vi "plot magnetotropic -- all.vi"() -> ()   [LabVIEW 2020]
uses:
  <vilib>/event_ctls.llb/eventvkey.ctl
  <vilib>/Analysis/baseanly.llb/A x Vector.vi
  <vilib>/Analysis/baseanly.llb/Complex A x B.vi
  Q -- check range -- i -- real.vi
  line -- complex.vi
  Q -- check range -- i -- integer.vi
  aggregator - v - real - atomic.vi
  Q - not nan -- real.vi
  Q - not nan -- integer.vi
  linear interpolation - real.vi
  <vilib>/Analysis/Matrix/Numeric/Conversions/Array To Matrix.vi
  <vilib>/Analysis/Matrix/Numeric/Conversions/Array To Matrix - RA2.vi
  <vilib>/Analysis/baseanly.llb/Inverse Matrix.vi
  <vilib>/Analysis/baseanly.llb/Real Inverse Matrix.vi
  <vilib>/Analysis/NI_AALBase.lvlib
panel:
  in  "Tab Control":enum32{"Page 1", "Page 2"}(tab)
  in  "max alpha":dbl=360.0 format="%#_13g"
  out "Plot angles":cluster{dbl[], dbl[]}[](graph)=[{[0.0, 3.6, 7.2, 10.8, 14.4, 18.0, 21.6, 25.2, 28.8, 32.4, 36.0, 39.6, 43.2, 46.800000000000004, 50.4, 54.0, 57.6, 61.2, 64.8, 68.4, 72.0, 75.60000000000001, 79.2, 82.8, 86.4, 90.0, 93.60000000000001, 97.2, 100.8, 104.4, 108.0, 111.60000000000001, 115.2, 118.8, 122.4, 126.0, 129.6, 133.20000000000002, 136.8, 140.4, 144.0, 147.6, 151.20000000000002, 154.8, 158.4, 162.0, 165.6, 169.20000000000002, 172.8, 176.4, 180.0, 183.6, 187.20000000000002, 190.8, 194.4, 198.0, 201.6, 205.20000000000002, 208.8, 212.4, 216.0, 219.6, 223.20000000000002, 226.8, 230.4, 234.0, 237.6, 241.20000000000002, 244.8, 248.4, 252.0, 255.6, 259.2, 262.8, 266.40000000000003, 270.0, 273.6, 277.2, 280.8, 284.40000000000003, 288.0, 291.6, 295.2, 298.8, 302.40000000000003, 306.0, 309.6, 313.2, 316.8, 320.40000000000003, 324.0, 327.6, 331.2, 334.8, 338.40000000000003, 342.0, 345.6, 349.2, 352.8, 356.40000000000003], [-313.48146927140203, -305.858243348933, -284.2953550420243, -252.19459672026446, -213.84280315872593, -173.21720232347388, -133.2937756788047, -95.90672651415247, -61.945212185027714, -31.65615222148574, -4.916123418277465, 18.574327400526585, 39.170983826139434, 57.2211441404977, 73.03368491463019, 86.86906141407903, 98.9396043298828, 109.4144526814921, 118.42604419322804, 126.07661803927712, 132.44403837415837, 137.5866937086247, 141.54744356495215, 144.3566756438778, 146.03456403347786, 146.59261453117998, 146.03456403347747, 144.35667564387575, 141.54744356495738, 137.58669370862123, 132.4440383741633, 126.07661803929162, 118.42604419322953, 109.4144526814938, 98.93960432990127, 86.86906141404705, 73.03368491462109, 57.22114414049983, 39.170983826133465, 18.574327400523742, -4.916123418274623, -31.65615222148702, -61.945212185040646, -95.90672651414792, -133.29377567881153, -173.2172023234709, -213.84280315872715, -252.19459672026204, -284.29535504202454, -305.8582433489345, -313.4814692714306, -305.85824334893397, -284.2953550420227, -252.19459672026284, -213.84280315872985, -173.21720232347118, -133.29377567881508, -95.90672651414764, -61.9452121850415, -31.65615222148702, -4.916123418278744, 18.5743274005182, 39.170983826133465, 57.22114414047297, 73.0336849146181, 86.86906141404975, 98.93960432989743, 109.41445268149444, 118.42604419322932, 126.07661803929105, 132.44403837416343, 137.58669370862128, 141.54744356495735, 144.35667564387546, 146.03456403347747, 146.59261453117998, 146.03456403347553, 144.3566756438778, 141.54744356495374, 137.58669370862498, 132.4440383741574, 126.07661803927712, 118.42604419322853, 109.41445268148918, 98.93960432988536, 86.86906141408315, 73.03368491460375, 57.2211441404977, 39.1709838261356, 18.574327400526585, -4.916123418277465, -31.656152221493272, -61.945212185025866, -95.90672651419283, -133.29377567880485, -173.21720232347545, -213.84280315872545, -252.19459672026517, -284.29535504202306, -305.85824334893294]}, {[0.0, 3.6, 7.2, 10.8, 14.4, 18.0, 21.6, 25.2, 28.8, 32.4, 36.0, 39.6, 43.2, 46.800000000000004, 50.4, 54.0, 57.6, 61.2, 64.8, 68.4, 72.0, 75.60000000000001, 79.2, 82.8, 86.4, 90.0, 93.60000000000001, 97.2, 100.8, 104.4, 108.0, 111.60000000000001, 115.2, 118.8, 122.4, 126.0, 129.6, 133.20000000000002, 136.8, 140.4, 144.0, 147.6, 151.20000000000002, 154.8, 158.4, 162.0, 165.6, 169.20000000000002, 172.8, 176.4, 180.0, 183.6, 187.20000000000002, 190.8, 194.4, 198.0, 201.6, 205.20000000000002, 208.8, 212.4, 216.0, 219.6, 223.20000000000002, 226.8, 230.4, 234.0, 237.6, 241.20000000000002, 244.8, 248.4, 252.0, 255.6, 259.2, 262.8, 266.40000000000003, 270.0, 273.6, 277.2, 280.8, 284.40000000000003, 288.0, 291.6, 295.2, 298.8, 302.40000000000003, 306.0, 309.6, 313.2, 316.8, 320.40000000000003, 324.0, 327.6, 331.2, 334.8, 338.40000000000003, 342.0, 345.6, 349.2, 352.8, 356.40000000000003], [-52.098103078947666, -64.89098767355117, -109.04888534951418, -194.42645181689528, -298.8059333429718, -335.9390833991341, -266.9407778689754, -169.02628156661706, -97.14690185514655, -50.71491152292708, -18.003664188575215, 7.871623107547521, 29.77997548820923, 48.851124152969874, 65.59614496908608, 80.3111497772457, 93.20434301282972, 104.4349357297611, 114.1270103434394, 122.37670334950465, 129.25744555823945, 134.82430138343324, 139.11757735713303, 142.16571872494595, 143.98751207706195, 144.5936246043267, 143.98751207706334, 142.16571872494666, 139.1175773571345, 134.8243013834304, 129.2574455582536, 122.37670334947296, 114.12701034343726, 104.4349357297638, 93.2043430128337, 80.31114977728095, 65.59614496910967, 48.85112415302615, 29.77997548822117, 7.871623107423034, -18.00366418848654, -50.71491152304105, -97.14690185523153, -169.02628156654373, -266.9407778689721, -335.93908339917783, -298.8059333429725, -194.42645181688215, -109.0488853495065, -64.89098767354592, -52.09810307894766, -64.89098767354581, -109.04888534950685, -194.42645181688349, -298.80593334297214, -335.93908339917874, -266.94077786899186, -169.0262815665497, -97.14690185522329, -50.71491152305839, -18.003664188560435, 7.87162310743895, 29.77997548822117, 48.85112415304576, 65.59614496911792, 80.31114977728436, 93.20434301282688, 104.43493572977161, 114.12701034343144, 122.37670334946948, 129.25744555825858, 134.82430138342897, 139.11757735713473, 142.16571872494666, 143.98751207706334, 144.59362460432672, 143.9875120770618, 142.16571872494595, 139.11757735713337, 134.82430138343773, 129.25744555823934, 122.37670334949264, 114.12701034342888, 104.43493572976237, 93.20434301284024, 80.31114977723888, 65.59614496908722, 48.851124152969874, 29.779975488203547, 7.871623107547521, -18.003664188575215, -50.71491152291799, -97.14690185517213, -169.02628156661962, -266.9407778689721, -335.93908339913344, -298.80593334296805, -194.42645181689522, -109.04888534951428, -64.89098767355122]}]
  out "weight -- one spin":dbl=-52.99873886913457
  out "weight -- bipartite":dbl=-50.9668248690652
  in  "field":dbl(slide)=100.0 scale=0.0..100.0
  out "Plot":cluster{dbl[], dbl[]}[](graph)=[{[0.0, 2.0, 4.0, 6.0, 8.0, 10.0, 12.0, 14.0, 16.0, 18.0, 20.0, 22.0, 24.0, 26.0, 28.0, 30.0, 32.0, 34.0, 36.0, 38.0, 40.0, 42.0, 44.0, 46.0, 48.0, 50.0, 52.0, 54.0, 56.0, 58.0, 60.0, 62.0, 64.0, 66.0, 68.0, 70.0, 72.0, 74.0, 76.0, 78.0, 80.0, 82.0, 84.0, 86.0, 88.0, 90.0, 92.0, 94.0, 96.0, 98.0, 100.0, 102.0, 104.0, 106.0, 108.0, 110.0, 112.0, 114.0, 116.0, 118.0, 120.0, 122.0, 124.0, 126.0, 128.0, 130.0, 132.0, 134.0, 136.0, 138.0, 140.0, 142.0, 144.0, 146.0, 148.0, 150.0, 152.0, 154.0, 156.0, 158.0, 160.0, 162.0, 164.0, 166.0, 168.0, 170.0, 172.0, 174.0, 176.0, 178.0, 180.0, 182.0, 184.0, 186.0, 188.0, 190.0, 192.0, 194.0, 196.0, 198.0], [0.0, 1.1385133282404225, 3.9788841114054527, 7.490878120034998, 11.038654301749444, 14.427008958566468, 17.658021528651247, 20.779726830573175, 23.83474181657537, 26.851283092850977, 29.845953470720342, 32.82793129135691, 35.802100017435976, 38.77099118470959, 41.73589205829657, 44.69744710271395, 47.655974462149786, 50.61162883821093, 53.56448394311787, 56.514573698509345, 59.46191264750393, 62.40650591614422, 65.34835410385297, 68.2874556359068, 71.22380789870721, 74.15740778407016, 77.0882519491738, 80.01633694023977, 82.94165925124416, 85.86421535166762, 88.78400169961012, 91.7010147479711, 94.61525094734984, 97.52670674741232, 100.43537859753108, 103.3412629471093, 106.24435624570754, 109.14465494316207, 112.04215548948886, 114.93685433509711, 117.82874793066647, 120.71783272722843, 123.60410517612117, 126.48756172904706, 129.36819883805785, 132.246012955557, 135.1210005343324, 137.99315802753523, 140.86248188871986, 143.72896857181993, 146.59261453117998, 149.4534162215584, 152.31137009813247, 155.1664726165046, 158.01872023271412, 160.86810940324898, 163.71463658505473, 166.5582982355258, 169.39909081253347, 172.23701077443422, 175.0720545800654, 177.9042186887598, 180.73349956035088, 183.5598936551813, 186.38339743413349, 189.2040073585988, 192.02171989050532, 194.83653149232848, 197.64843862711643, 200.45743775844693, 203.2635253504933, 206.0666978679967, 208.86695177628366, 211.66428354127544, 214.45868962950044, 217.2501665080932, 220.03871064481868, 222.82431850806068, 225.60698656683422, 228.38671129080834, 231.1634891502969, 233.937316616298, 236.70819016043666, 239.4761062550522, 242.24106137315607, 245.003051988445, 247.7620745753361, 250.51812560894987, 253.27120156510438, 256.02129892038096, 258.7684141520641, 261.5125437382003, 264.2536841575947, 266.9918318897845, 269.7269834150807, 272.4591352145985, 275.1882837702045, 277.9144255645732, 280.637557081188, 283.3576748043006]}, {[0.0, 2.0, 4.0, 6.0, 8.0, 10.0, 12.0, 14.0, 16.0, 18.0, 20.0, 22.0, 24.0, 26.0, 28.0, 30.0, 32.0, 34.0, 36.0, 38.0, 40.0, 42.0, 44.0, 46.0, 48.0, 50.0, 52.0, 54.0, 56.0, 58.0, 60.0, 62.0, 64.0, 66.0, 68.0, 70.0, 72.0, 74.0, 76.0, 78.0, 80.0, 82.0, 84.0, 86.0, 88.0, 90.0, 92.0, 94.0, 96.0, 98.0, 100.0, 102.0, 104.0, 106.0, 108.0, 110.0, 112.0, 114.0, 116.0, 118.0, 120.0, 122.0, 124.0, 126.0, 128.0, 130.0, 132.0, 134.0, 136.0, 138.0, 140.0, 142.0, 144.0, 146.0, 148.0, 150.0, 152.0, 154.0, 156.0, 158.0, 160.0, 162.0, 164.0, 166.0, 168.0, 170.0, 172.0, 174.0, 176.0, 178.0, 180.0, 182.0, 184.0, 186.0, 188.0, 190.0, 192.0, 194.0, 196.0, 198.0], [0.0, 8.900130425564837e-10, 4.980541071344847e-09, 1.8027194455800313e-08, 5.5968542752720894e-08, 1.603846822900161e-07, 4.3714180784073774e-07, 1.1513864569353502e-06, 2.9587779768584587e-06, 7.464085178354467e-06, 1.8562061001715787e-05, 4.5638678412783686e-05, 0.00011117792754096806, 0.0002687627106131862, 0.0006455171293070279, 0.00154184819773502, 0.0036651375561248143, 0.008675688934056123, 0.020458309058919093, 0.04807318354057271, 0.11256725639316362, 0.2625492229354917, 0.609136878749996, 1.401214132611615, 3.1726654095564144, 6.965349415930417, 14.418812324214018, 26.980292311505405, 43.74223661144523, 60.66714990650701, 74.0508267865482, 83.2603048838894, 89.49849983930051, 94.05036922442446, 97.74224194918389, 101.01638492343656, 104.09155006689397, 107.0721685756904, 110.00728703682107, 112.91976128369079, 115.8202004532285, 118.71351867786251, 121.60198947594043, 124.48666403616657, 127.36802830740446, 130.24630699257403, 133.12160404575195, 135.99396755810986, 138.8634197099153, 141.72997059496893, 144.5936246043267, 147.45438337876269, 150.3122471791845, 153.16721552756238, 156.0192875109634, 158.86846192981622, 161.71473737360589, 164.5581122624082, 167.39858487224797, 170.2361533521153, 173.07081573690914, 175.9025699578329, 178.73141385126098, 181.55734516654846, 184.3803615729486, 187.2004606659003, 190.01763997262435, 192.83189695733006, 195.64322902584985, 198.45163352995888, 201.2571077712471, 204.0596490047167, 206.85925444206575, 209.65592125469044, 212.4496465764564, 215.2404275062642, 218.02826111037606, 220.81314442459785, 223.59507445624843, 226.37404818606007, 229.15006256984785, 231.9231145401189, 234.6932010075055, 237.460318862166, 240.2244649750537, 242.9856361990703, 245.74382937016685, 248.49904130838834, 251.25126881880405, 254.0005086923912, 256.7467577068962, 259.4900126275882, 262.2302702079803, 264.96752719051915, 267.70178030720695, 270.433026280264, 273.16126182257307, 275.88648363830816, 278.6086884233937, 281.32787286592304]}, {[0.0, 2.0, 4.0, 6.0, 8.0, 10.0, 12.0, 14.0, 16.0, 18.0, 20.0, 22.0, 24.0, 26.0, 28.0, 30.0, 32.0, 34.0, 36.0, 38.0, 40.0, 42.0, 44.0, 46.0, 48.0, 50.0, 52.0, 54.0, 56.0, 58.0, 60.0, 62.0, 64.0, 66.0, 68.0, 70.0, 72.0, 74.0, 76.0, 78.0, 80.0, 82.0, 84.0, 86.0, 88.0, 90.0, 92.0, 94.0, 96.0, 98.0, 100.0, 102.0, 104.0, 106.0, 108.0, 110.0, 112.0, 114.0, 116.0, 118.0, 120.0, 122.0, 124.0, 126.0, 128.0, 130.0, 132.0, 134.0, 136.0, 138.0, 140.0, 142.0, 144.0, 146.0, 148.0, 150.0, 152.0, 154.0, 156.0, 158.0, 160.0, 162.0, 164.0, 166.0, 168.0, 170.0, 172.0, 174.0, 176.0, 178.0, 180.0, 182.0, 184.0, 186.0, 188.0, 190.0, 192.0, 194.0, 196.0, 198.0], [4.1407275882666, 6.99010825547407, 9.83948892268154, 12.68886958988901, 15.538250257096479, 18.38763092430395, 21.23701159151142, 24.086392258718888, 26.935772925926358, 29.785153593133828, 32.6345342603413, 35.48391492754877, 38.33329559475624, 41.18267626196371, 44.032056929171176, 46.881437596378646, 49.730818263586116, 52.580198930793586, 55.429579598001055, 58.278960265208525, 61.128340932415995, 63.977721599623464, 66.82710226683093, 69.6764829340384, 72.52586360124587, 75.37524426845334, 78.22462493566081, 81.07400560286828, 83.92338627007575, 86.77276693728322, 89.62214760449069, 92.47152827169816, 95.32090893890563, 98.1702896061131, 101.01967027332057, 103.86905094052804, 106.71843160773551, 109.56781227494298, 112.41719294215045, 115.26657360935792, 118.11595427656539, 120.96533494377286, 123.81471561098033, 126.6640962781878, 129.51347694539527, 132.36285761260274, 135.2122382798102, 138.06161894701768, 140.91099961422515, 143.76038028143262, 146.6097609486401, 149.45914161584756, 152.30852228305503, 155.1579029502625, 158.00728361746997, 160.85666428467744, 163.7060449518849, 166.55542561909238, 169.40480628629984, 172.25418695350731, 175.10356762071478, 177.95294828792225, 180.80232895512972, 183.6517096223372, 186.50109028954466, 189.35047095675213, 192.1998516239596, 195.04923229116707, 197.89861295837454, 200.747993625582, 203.59737429278948, 206.44675495999695, 209.29613562720442, 212.1455162944119, 214.99489696161936, 217.84427762882683, 220.6936582960343, 223.54303896324177, 226.39241963044924, 229.2418002976567, 232.09118096486418, 234.94056163207165, 237.78994229927912, 240.6393229664866, 243.48870363369406, 246.33808430090153, 249.187464968109, 252.03684563531647, 254.88622630252394, 257.7356069697314, 260.5849876369389, 263.43436830414635, 266.2837489713538, 269.1331296385613, 271.98251030576876, 274.8318909729762, 277.6812716401837, 280.53065230739116, 283.38003297459863, 286.2294136418061]}]
  in  "g":dbl[](array[numeric])=[2.0, 2.0, 1.0]
  in  "theta v":dbl(slide)=90.0 scale=0.0..180.0
  in  "phi v":dbl(slide)=90.0 scale=-180.0..180.0
  in  "theta r":dbl(slide)=90.0 scale=0.0..180.0
  in  "phi r":dbl(slide)=90.0 scale=-180.0..180.0
  in  "theta 0":dbl(slide) scale=0.0..180.0
  in  "phi 0":dbl(slide)=41.53846153846155 scale=-180.0..180.0
  in  "nsteps":i32=100
  in  "integration nsteps":i32=300
  in  "scale":dbl(slide)=175.50446715591082 scale=0.01..200.0
  in  "alpha":dbl(slide)=90.0 scale=0.0..180.0
  in  "temperature":dbl(slide)=10.0 scale=0.0..300.0
  in  "max B":dbl=200.0 format="%#_13g"
  in  "JR":dbl(slide)=30.0 scale=-100.0..100.0
  out "Plot slope":cluster{dbl[], dbl[]}[](graph)=[{[171.0, 153.0, 135.0, 117.0, 99.0, 81.0, 63.0, 44.999999999999986, 27.000000000000007, 9.0, 11.0, 13.0, 15.0, 17.0, 19.0, 21.0, 23.0, 25.0, 27.0, 29.0, 31.0, 33.0, 35.0, 37.0, 39.0, 41.0, 43.0, 45.0, 47.0, 49.0, 51.0, 53.0, 55.0, 57.0, 59.0, 61.0, 63.0, 65.0, 67.0, 69.0, 71.0, 73.0, 75.0, 77.0, 79.0, 81.0, 83.0, 85.0, 87.0, 89.0, 91.0, 93.0, 95.0, 97.0, 99.0, 101.0, 103.0, 105.0, 107.0, 109.0, 111.0, 113.0, 115.0, 117.0, 119.0, 121.0, 123.0, 125.0, 127.0, 129.0, 131.0, 133.0, 135.0, 137.0, 139.0, 141.0, 143.0, 145.0, 147.0, 149.0, 151.0, 153.0, 155.0, 157.0, 159.0, 161.0, 163.0, 165.0, 167.0, 169.0, 171.0, 173.0, 175.0, 177.0, 179.0, 181.0, 183.0, 185.0, 187.0, 189.0], [1.4334395824795205, 1.4378984361647174, 1.4391915931880157, 1.4388213190853891, 1.437759503777789, 1.4365055311326125, 1.4352873811607882, 1.4342395827903722, 1.4336906283992634, 1.5709974113106284, 1.6140827357324117, 1.5955606057752005, 1.560774115888579, 1.5311558768756761, 1.511081334019714, 1.4986777642293596, 1.4912045223710173, 1.486591104266278, 1.4835445248733947, 1.4813260593728472, 1.4795343923153226, 1.4779584134129422, 1.476489526712598, 1.4750727868475906, 1.4736807472015983, 1.4722998371799036, 1.4709234031492002, 1.4695482057312574, 1.468172677249612, 1.4667960626977958, 1.4654180004614545, 1.4640383178799539, 1.4626569328606536, 1.4612738065267479, 1.459888920553027, 1.4585022663597158, 1.4571138399768984, 1.4557236396114774, 1.45433166449493, 1.4529379143440337, 1.4515423891041053, 1.4501450888305385, 1.4487460136319328, 1.4473451636438313, 1.4459425390166984, 1.4445381399100938, 1.443131966490398, 1.441724018930131, 1.4403142974046546, 1.438902802094617, 1.4374895331849302, 1.436074490864712, 1.434657675327344, 1.4332390867704135, 1.4318187253955443, 1.4303965914083392, 1.428972685019346, 1.4275470064425804, 1.426119555896662, 1.4246903336037349, 1.4232593397910023, 1.4218265746894758, 1.4203920385339188, 1.418955731563642, 1.417517654022049, 1.416077806157091, 1.4146361882203564, 1.4131928004674137, 1.4117476431589466, 1.4103007165584813, 1.4088520209347735, 1.4074015565603304, 1.4059493237123206, 1.404495322671096, 1.403039553720987, 1.40158201715235, 1.4001227132580425, 1.3986616423355827, 1.3971988046858996, 1.3957342006146973, 1.3942678304321134, 1.3927996944523784, 1.3913297929934743, 1.3898581263767937, 1.388384694929755, 1.3869094989825044, 1.3854325388692814, 1.3839538149291002, 1.3824733275046128, 1.3809910769427916, 1.3795070635940192, 1.3780212878139082, 1.3765337499621637, 1.3750444504016741, 1.3735533895001026, 1.3720605676287505, 1.3705659851627843, 1.3690696424832822, 1.3675715399729143, 1.366071678020262]}, {[171.0, 153.0, 135.0, 117.0, 99.0, 81.0, 63.0, 44.999999999999986, 27.000000000000007, 9.0, 11.0, 13.0, 15.0, 17.0, 19.0, 21.0, 23.0, 25.0, 27.0, 29.0, 31.0, 33.0, 35.0, 37.0, 39.0, 41.0, 43.0, 45.0, 47.0, 49.0, 51.0, 53.0, 55.0, 57.0, 59.0, 61.0, 63.0, 65.0, 67.0, 69.0, 71.0, 73.0, 75.0, 77.0, 79.0, 81.0, 83.0, 85.0, 87.0, 89.0, 91.0, 93.0, 95.0, 97.0, 99.0, 101.0, 103.0, 105.0, 107.0, 109.0, 111.0, 113.0, 115.0, 117.0, 119.0, 121.0, 123.0, 125.0, 127.0, 129.0, 131.0, 133.0, 135.0, 137.0, 139.0, 141.0, 143.0, 145.0, 147.0, 149.0, 151.0, 153.0, 155.0, 157.0, 159.0, 161.0, 163.0, 165.0, 167.0, 169.0, 171.0, 173.0, 175.0, 177.0, 179.0, 181.0, 183.0, 185.0, 187.0, 189.0], [1.4228505873489876, 1.4302298287268371, 1.4373980657259202, 1.4444417765713755, 1.4513353356593486, 1.4579895421441122, 1.4641821113997207, 1.4692400559584013, 1.4698156493032637, 2.878053694270109e-07, 7.197910186034931e-07, 1.7777621975970876e-06, 4.346711137689153e-06, 1.0540086340924848e-05, 2.538109110851928e-05, 6.075908336659327e-05, 0.00014471062995128492, 0.00034312708036593974, 0.0008103750075541928, 0.0019069342321733984, 0.004471485258297419, 0.010445242808688561, 0.024282644800160916, 0.05603634168776467, 0.12762432660963208, 0.2834546627868457, 0.60042714206112, 1.1727879291458843, 2.039221062520628, 3.103182761562259, 4.166915288712467, 5.038704135401218, 5.589161792668008, 5.751440505502984, 5.5119450013245626, 4.915018157022303, 4.080401940802631, 3.2023201820192355, 2.47761327451218, 1.9948948931163955, 1.7207194676356323, 1.579287605061097, 1.5097040882571946, 1.4759558896506064, 1.4593903843470457, 1.4509112674280118, 1.4462038048068848, 1.4432477580957652, 1.4411031491842436, 1.4393340231053458, 1.4377385283193576, 1.4362232794082388, 1.4347450716511503, 1.433283893868122, 1.4318304489680145, 1.430380388611752, 1.428931651602511, 1.4274832357432388, 1.4260346312472052, 1.4245855592653243, 1.423135851076836, 1.4216853921062693, 1.420234095824867, 1.4187818914391528, 1.41732871795341, 1.4158745211948371, 1.4144192522244339, 1.412962866408634, 1.4115053228207444, 1.4100465838032505, 1.4085866146300532, 1.4071253832229331, 1.405662859907011, 1.4041990171976977, 1.4027338296092466, 1.4012672734867238, 1.3997993268499158, 1.3983299692563378, 1.396859181675154, 1.3953869463746287, 1.3939132468198068, 1.392438067578155, 1.3909613942350916, 1.3894832133162254, 1.388003512216983, 1.3865222791378073, 1.3850395030276559, 1.383555173526247, 1.3820692809165394, 1.3805818160794843, 1.3790927704530986, 1.3776021359938113, 1.3761099051400834, 1.3746160707814852, 1.3731206262257274, 1.3716235651777424, 1.3701248817067153, 1.3686245702272117, 1.3671226254764406, 1.3656190424931083]}]
  in  "JO":dbl(slide)=25.0 scale=-100.0..100.0
  in  "JK":dbl(slide) scale=-100.0..100.0
  in  "slope win":i32=10
  in  "G1":dbl(slide) scale=-10.0..10.0
  in  "G2":dbl(slide) scale=-10.0..10.0
  in  "G3":dbl(slide) scale=-10.0..10.0
  in  "slope B":dbl(slide)=90.0 scale=0.0..200.0
  in  "slope delta B":dbl(slide)=10.0 scale=0.0..20.0
  in  "spins":enum16{"spin one half", "bipartite"}(ring)
  in  "B":dbl=5.0 format="%#_13g"
  in  "jj":dbl[](array[numeric])=[0.0, 0.0]
  in  "save?":bool
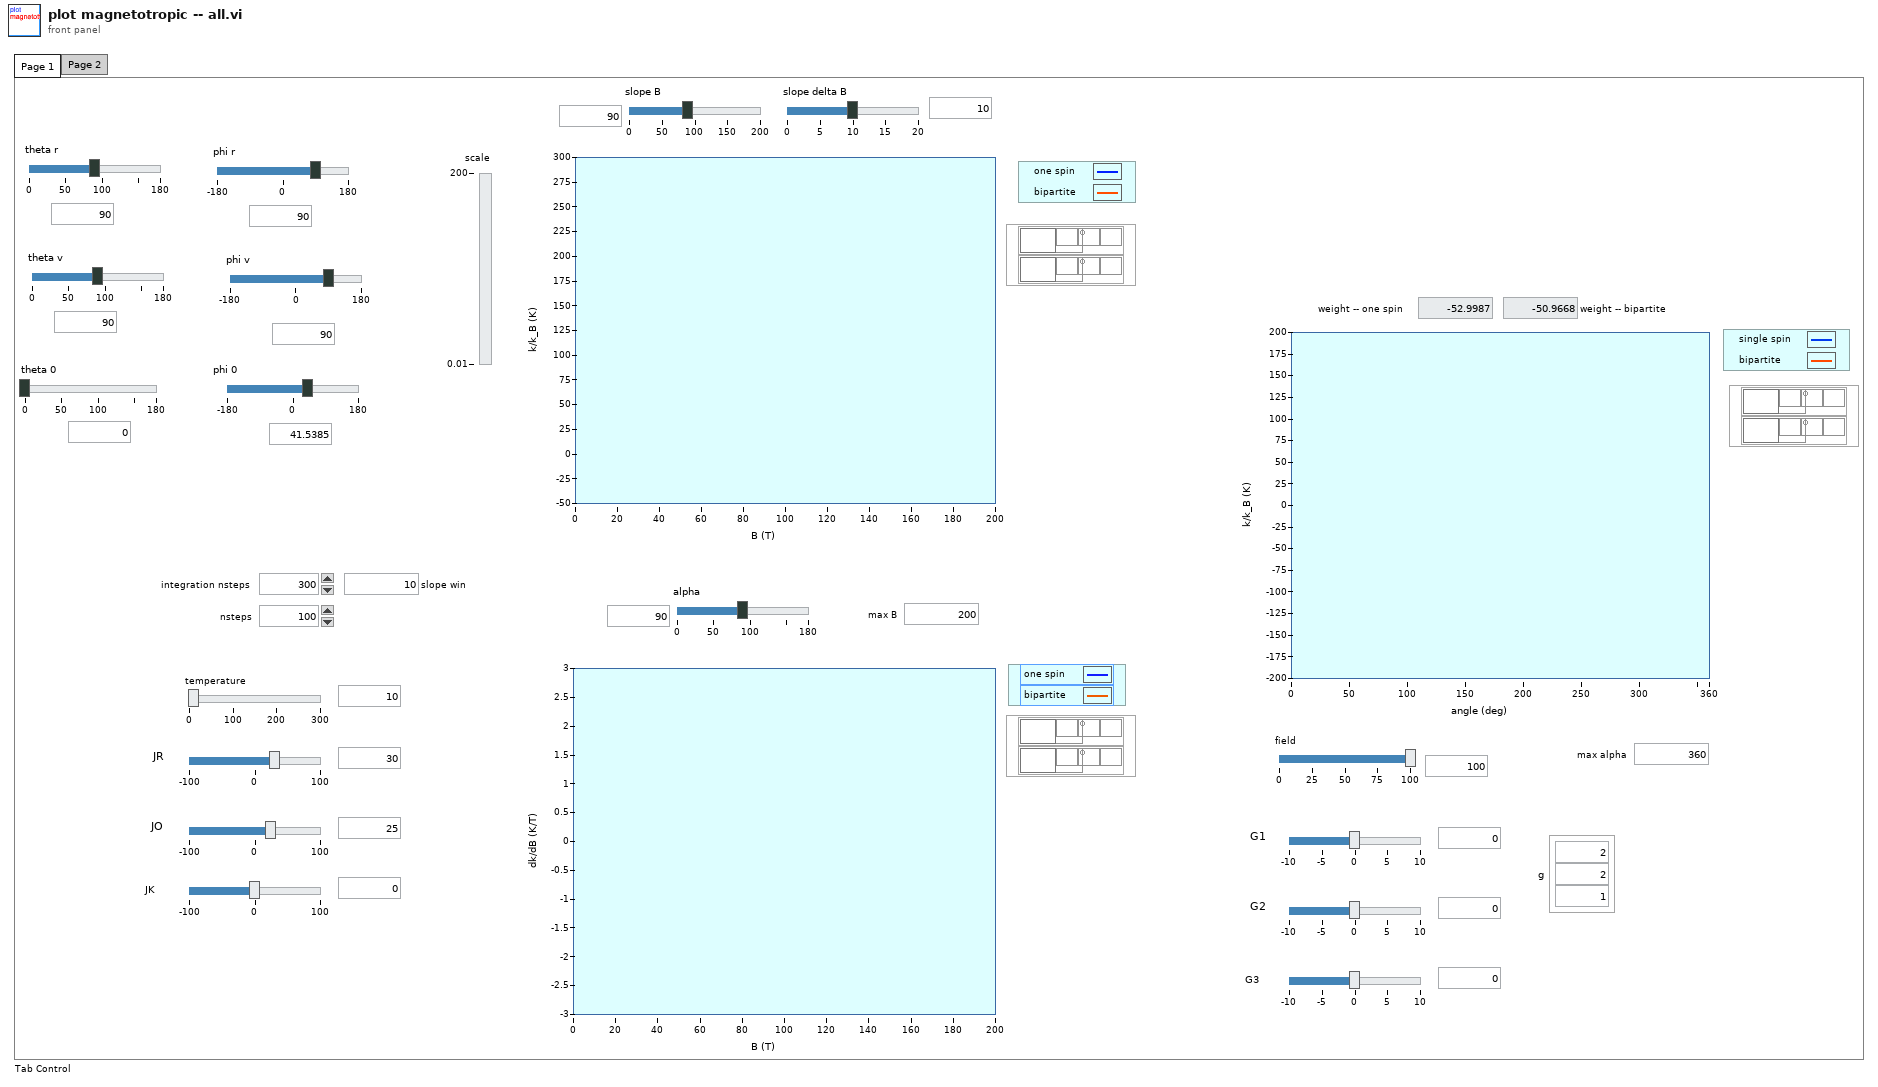
[diagram p1: front panel]
types:
  T1 = typedef "eventvkey.ctl" = enum16{"ASCII", "Enter", "Return", "Shift", "Ctrl", "Alt", "Cmd", "Opt", "Caps", "NumLock", "Clear", "Break", "Up", "Down", "Left", "Right", "Insert", "Delete", "Home", "End", "PageUp", "PageDown", "Escape", "Help", "Pause", "ScrollLock", "F1", "F2", "F3", "F4", "F5", "F6", "F7", "F8", "F9", "F10", "F11", "F12", "F13", "F14", "F15", "F16", "F17", "F18", "F19", "F20", "F21", "F22", "F23", "F24", "Play", "VolumeUp", "VolumeDown", "Mute", "Two Byte Char"}
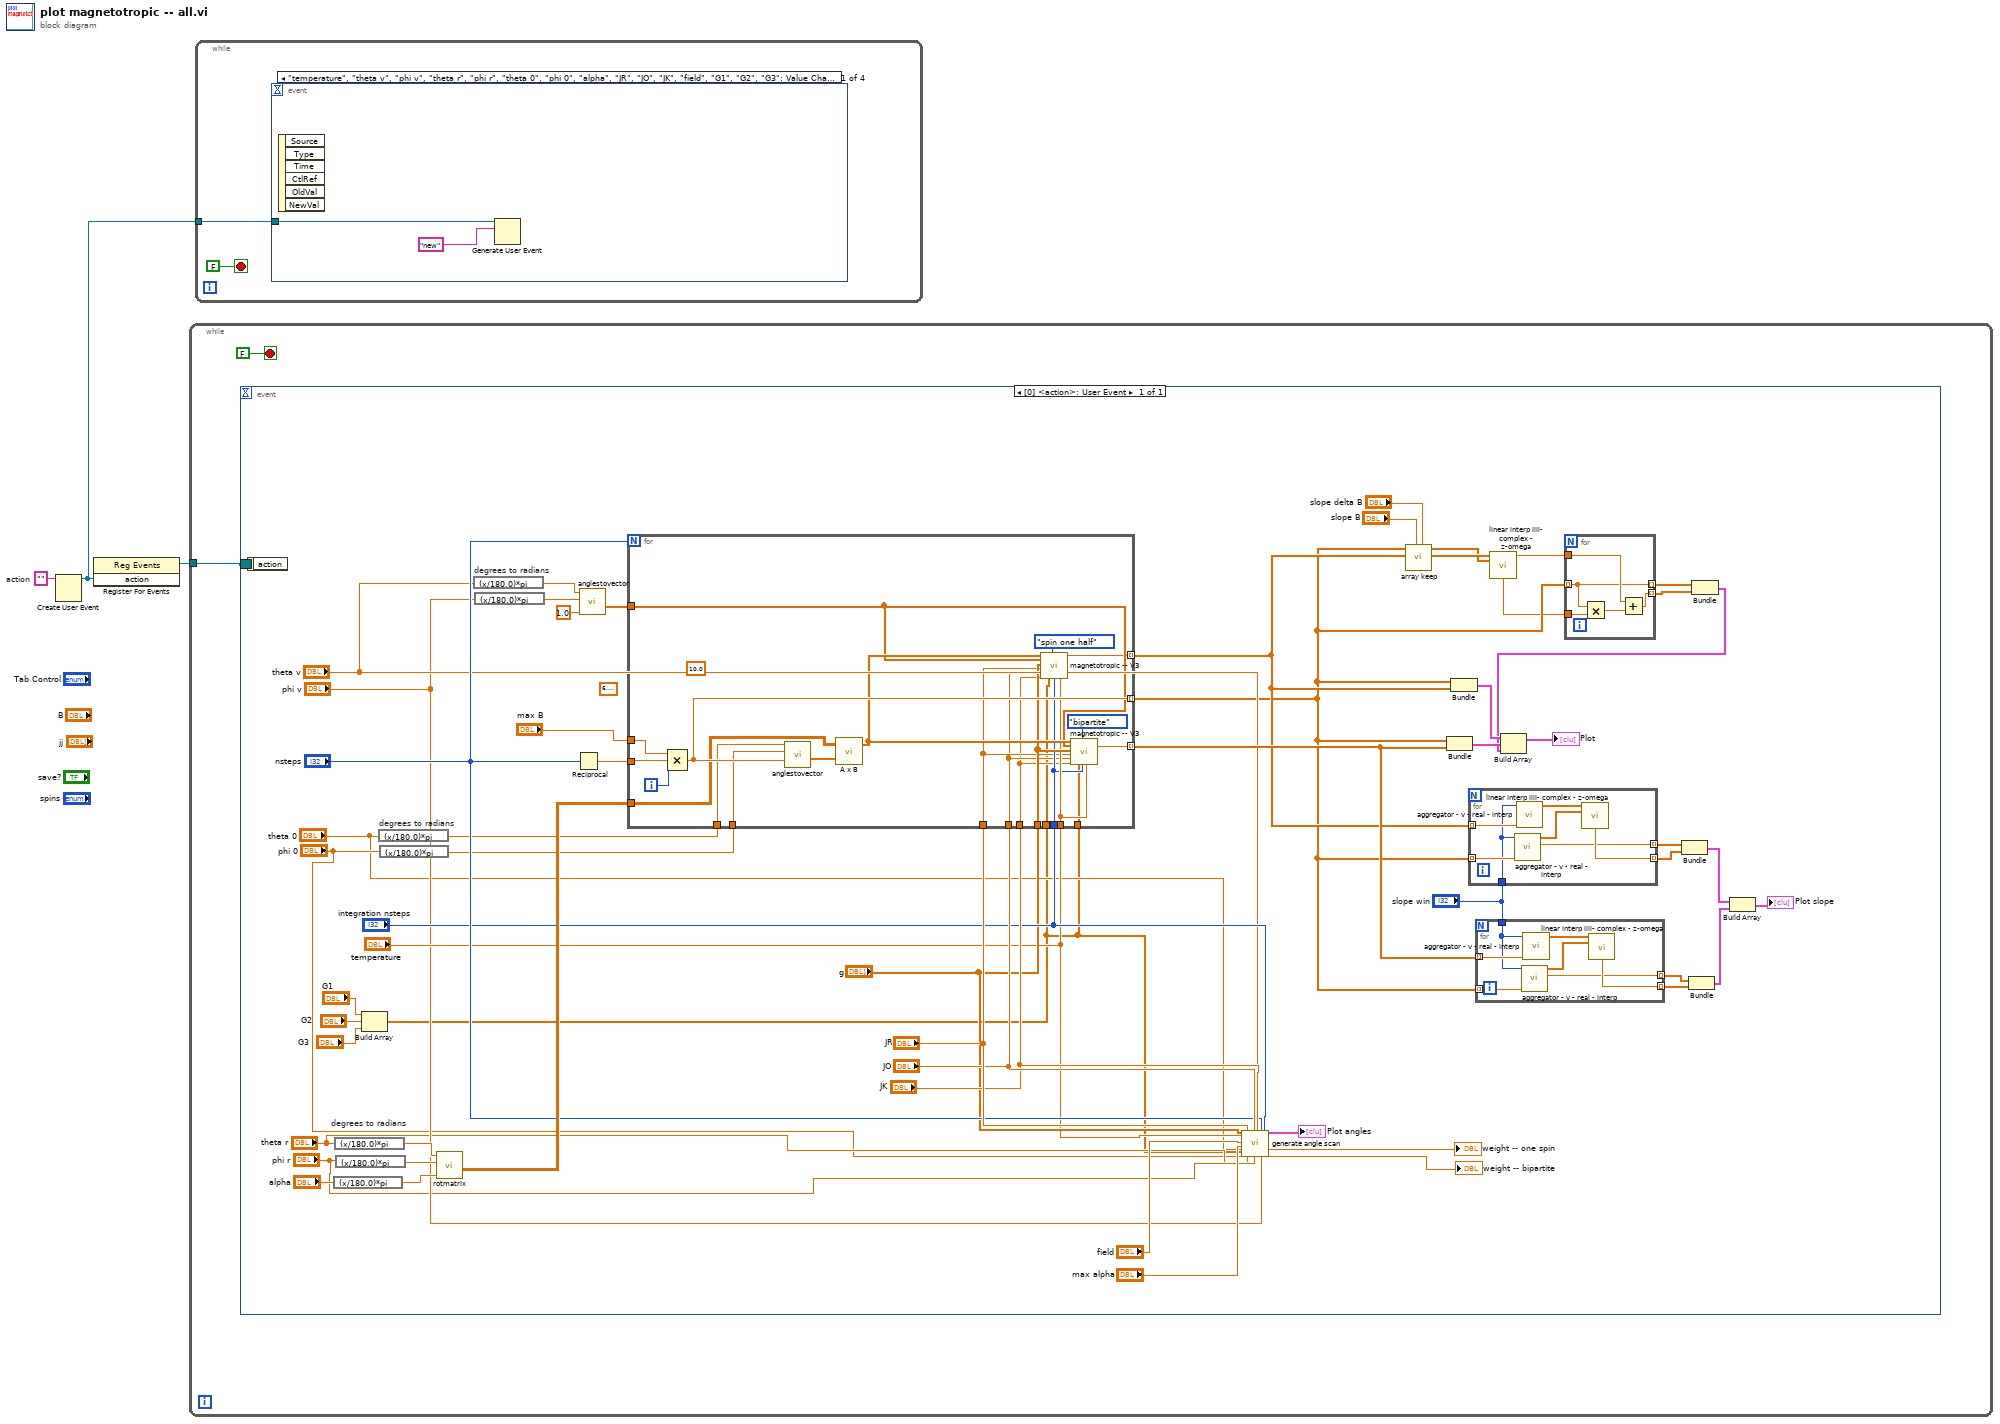
[diagram p0: block diagram]
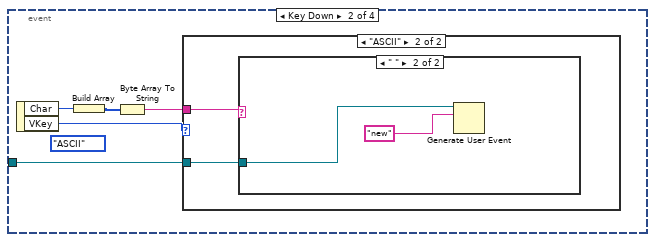
[diagram p2: hidden frame]
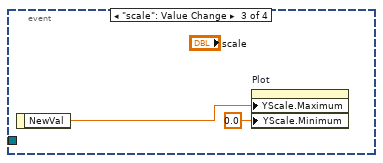
[diagram p5: hidden frame]
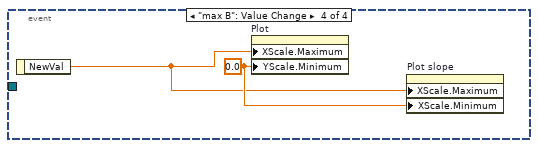
[diagram p6: hidden frame]
diagram:
  w2 = ""  # action
  n1 = Create User Event(user event datatype=w2) -> (user event=w1:refnum<user-event>)  [unwired: 1 in, 1 out]
  n2 = register-events(w1) -> (reference out=w3:refnum<event-registration>)  [unwired: 2 in, 1 out]
  n3 = while {
    tunnel: w3 -> [w5]
    stop <- FALSE stop-if-true
    n4 = event shown="[0] <action>: User Event" {
      selector: w5 -> [_]
      dyn-events: _ -> [_]
      timeout: _ -> [_]
      event User Event {
        (unwired) 6.283185307179586
        n5 = event-data() -> ()  [unwired: 1 in, 1 out]
        n6 = expression code="(x/180.0)*pi" ("degrees to radians")("alpha") -> (w55:dbl)
        n7 = expression code="(x/180.0)*pi" "degrees to radians"("theta r") -> (w54:dbl)
        n8 = expression code="(x/180.0)*pi" ("degrees to radians")("phi r") -> (w53:dbl)
        n9 = Build Array("G1", "G2", "G3") -> (w17:dbl[])
        n10 = expression code="(x/180.0)*pi" "degrees to radians"("theta 0") -> (w27:dbl)
        n11 = expression code="(x/180.0)*pi" ("degrees to radians")("phi 0") -> (w28:dbl)
        n12 = call "rotmatrix.vi"("alpha"=w55, "phi"=w53, "theta"=w54) -> ("matr"=w52:dbl[][])  [unwired: 8 in]
        n13 = expression code="(x/180.0)*pi" "degrees to radians"("theta v") -> (w59:dbl)
        n14 = expression code="(x/180.0)*pi" ("degrees to radians")("phi v") -> (w60:dbl)
        n15 = Reciprocal(x="nsteps") -> (1/x=w62:dbl)
        n16 = call "anglestovector.vi"("R"=1.0, "phi"=w60, "theta"=w59) -> ("B"=w57:dbl[])  [unwired: 8 in]
        n17 = for {
          N: "nsteps" -> [_]
          tunnel: w62 -> [w103]
          tunnel: [w98] -> w50 mode=indexing
          tunnel: [w101] -> w11 mode=indexing
          tunnel: "max B" -> [w100]
          tunnel: "integration nsteps" -> [w90]
          tunnel: "g" -> [w95]
          tunnel: "temperature" -> [w91]
          tunnel: w57 -> [w96]
          tunnel: w52 -> [w99]
          tunnel: [w92] -> w14 mode=indexing
          tunnel: "JR" -> [w89]
          tunnel: "JO" -> [w88]
          tunnel: "JK" -> [w87]
          tunnel: w28 -> [w86]
          tunnel: w27 -> [w85]
          tunnel: w17 -> [w84]
          tunnel: w17 -> [w83]
          i -> [w104]
          (unwired) 10.0 ("value")
          n18 = Compound Arithmetic op=MULTIPLY(w100, w103, w104) -> (w101:dbl)
          n19 = call "anglestovector.vi"("R"=w101, "phi"=w86, "theta"=w85) -> ("B"=w102:dbl[])  [unwired: 8 in]
          n20 = call-poly <vilib>:"A x B.vi"("Vector"=w102, "A"=w99) -> ("A x Vector"=w97:dbl[])  [unwired: 1 out]
          n21 = call "magnetotropic -- V3.vi"("B"=w97, "n"=w96, "g"=w95, "JR"=w89, "JO"=w88, "JK"=w87, "G"=w84, "spins"=enum16{"spin one half", "bipartite"}."spin one half", "nsteps"=w90, "temperature"=w91) -> ("magnetotropic"=w92:dbl)  [unwired: 9 in]
          n22 = call "magnetotropic -- V3.vi"("B"=w97, "n"=w96, "g"=w95, "JR"=w89, "JO"=w88, "JK"=w87, "G"=w83, "spins"=enum16{"spin one half", "bipartite"}."bipartite", "nsteps"=w90, "temperature"=w91) -> ("magnetotropic"=w98:dbl)  [unwired: 9 in]
        }
        n23 = call "generate angle scan.vi"("g"="g", "temperature"="temperature", "field"="field", "max alpha"="max alpha", "theta 0"="theta 0", "phi 0"="phi 0", "JR"="JR", "theta r"="theta r", "G"=w17, "JO"="JO", "phi r"="phi r", "JK"="JK", "theta v"="theta v", "nsteps"="nsteps", "phi v"="phi v", "integration nsteps"="integration nsteps") -> ("Plot"=→"Plot angles":cluster{dbl[], dbl[]}[], "weight -- one spin"=→"weight -- one spin":dbl, "weight -- bipartite"=→"weight -- bipartite":dbl)  [unwired: 9 in]
        n24 = call "array keep.vi"("slope win"="slope delta B", "slope B"="slope B", "Y"=w14, "X"=w11) -> ("Y out"=w13:dbl[], "X out"=w12:dbl[])  [unwired: 6 in]
        n25 = Bundle(w11, w50) -> (w48:cluster{dbl[], dbl[]})  [unwired: 1 in]
        n26 = Bundle(w11, w14) -> (w49:cluster{dbl[], dbl[]})  [unwired: 1 in]
        n27 = for {
          tunnel: w14 -> [w75] mode=indexing
          tunnel: w11 -> [w74] mode=indexing
          tunnel: [w71] -> w43 mode=indexing
          tunnel: [w70] -> w44 mode=indexing
          tunnel: "slope win" -> [w69]
          n28 = call "aggregator - v - real - interp.vi"("number"=w74, "requested size"=w69) -> ("mean"=w70:dbl, "Array"=w72:dbl[])  [unwired: 6 in, 2 out]
          n29 = call "aggregator - v - real - interp.vi"("number"=w75, "requested size"=w69) -> ("Array"=w73:dbl[])  [unwired: 6 in, 3 out]
          n30 = call "linear interp iiii- complex - z-omega.vi"("z"=w73, "omega"=w72) -> ("slope"=w71:cdb)  [unwired: 5 in, 8 out]
        }
        n31 = for {
          tunnel: w50 -> [w82] mode=indexing
          tunnel: w11 -> [w81] mode=indexing
          tunnel: [w78] -> w51 mode=indexing
          tunnel: [w77] -> w61 mode=indexing
          tunnel: "slope win" -> [w76]
          n32 = call "aggregator - v - real - interp.vi"("number"=w81, "requested size"=w76) -> ("mean"=w77:dbl, "Array"=w79:dbl[])  [unwired: 6 in, 2 out]
          n33 = call "aggregator - v - real - interp.vi"("number"=w82, "requested size"=w76) -> ("Array"=w80:dbl[])  [unwired: 6 in, 3 out]
          n34 = call "linear interp iiii- complex - z-omega.vi"("z"=w80, "omega"=w79) -> ("slope"=w78:cdb)  [unwired: 5 in, 8 out]
        }
        n35 = call "linear interp iiii- complex - z-omega.vi"("z"=w13, "omega"=w12) -> ("intercept"=w9:cdb, "slope"=w10:cdb)  [unwired: 5 in, 7 out]
        n36 = for {
          tunnel: w11 -> [w64] mode=indexing
          tunnel: w10 -> [w68]
          tunnel: w9 -> [w67]
          tunnel: [w65] -> w7 mode=indexing
          tunnel: [w64] -> w8 mode=indexing
          n37 = Multiply(x=w64, y=w68) -> (x*y=w66:cdb)
          n38 = Add(x=w67, y=w66) -> (x+y=w65:cdb)
        }
        n39 = Bundle(w44, w43) -> (w45:cluster{dbl[], cdb[]})  [unwired: 1 in]
        n40 = Bundle(w61, w51) -> (w42:cluster{dbl[], cdb[]})  [unwired: 1 in]
        n41 = Bundle(w8, w7) -> (w6:cluster{dbl[], cdb[]})  [unwired: 1 in]
        n42 = Build Array(w49, w48, w6) -> (→"Plot":cluster{dbl[], cdb[]}[])
        n43 = Build Array(w45, w42) -> (→"Plot slope":cluster{dbl[], cdb[]}[])
      }
    }
  }
  n44 = while {
    tunnel: w1 -> [w105]
    stop <- FALSE stop-if-true
    n45 = event shown="[0] \"temperature\", \"theta v\", \"phi v\", \"theta r\", \"phi r\", \"theta 0\", \"phi 0\", \"alpha\", \"JR\", \"JO\", \"JK\", \"field\", \"G1\", \"G2\", \"G3\": Value Change" {
      selector: _ -> [_ _ _ _]
      dyn-events: _ -> [_ _ _ _]
      timeout: _ -> [_ _ _ _]
      tunnel: w105 -> [w108 w109 _ _]
      event "temperature", "theta v", "phi v", "theta r", "phi r", "theta 0", "phi 0", "alpha", "JR", "JO", "JK", "field", "G1", "G2", "G3": Value Change {
        n46 = event-data() -> ()  [unwired: 1 in, 6 out]
        n47 = Generate User Event(user event=w108, event data cluster="new" ("event data")) -> ()  [unwired: 2 in, 2 out]
      }
      event Key Down {
        (unwired) eventvkey."ASCII" ("VKey")
        n48 = event-data() -> ("Char"=w112:i16, "VKey"=w111:T1)  [unwired: 1 in]
        n49 = Build Array(w112) -> (w113:i16[])
        n50 = Byte Array To String(unsigned byte array=w113) -> (string=w110:string)
        n51 = case shown="\"ASCII\"" w111 {
          tunnel: w110 -> [_ w115]
          tunnel: w109 -> [_ w114]
          frame "Escape", Default {
          }
          frame "ASCII" {
            n52 = case shown="\" \"" w115 {
              tunnel: w114 -> [_ w116]
              frame "False", Default {
              }
              frame " " {
                n53 = Generate User Event(user event=w116, event data cluster="new" ("event data")) -> ()  [unwired: 2 in, 2 out]
              }
            }
          }
        }
      }
      event "scale": Value Change {
        n54 = event-data() -> ("NewVal"=w119:dbl)  [unwired: 1 in]
        n55 = property on="Plot" class="XYGraph (strict)"("YScale.Maximum"=w119, "YScale.Minimum"=0.0 ("Y Scale.Range:Minimum")) -> ()  [unwired: 2 in, 2 out]
      }
      event "max B": Value Change {
        w121 = 0.0 ("Y Scale.Range:Minimum")
        n56 = event-data() -> ("NewVal"=w120:dbl)  [unwired: 1 in]
        n57 = property on="Plot" class="XYGraph (strict)"("XScale.Maximum"=w120, "YScale.Minimum"=w121) -> ()  [unwired: 2 in, 2 out]
        n58 = property on="Plot slope" class="XYGraph (strict)"("XScale.Maximum"=w120, "XScale.Minimum"=w121) -> ()  [unwired: 2 in, 2 out]
      }
    }
  }
